vi "SERIAL_Close.vi"(11 "navX DevRef":T1={"SerialPortRef"={"DevStatus"={"status"=FALSE, "code"=0, "source"=""}, "Serial Port Name"=""}, "Board Information"={"WhoAmI (50 | 0x32)"=0, "Board Revision"=0, "Firmware Major Version"=0, "Firmware Minor Version"=0}, "Status"={"Update Rate Hz"=0, "Accelerometer Full-Scale Range"=0, "Gyro Full-Scale Range"=0, "NAVX_OP_STATUS"=0, "NAVX_CAL_STATUS"=0, "NAVX_SELFTEST_STATUS"=0, "NAVX_SENSOR_STATUS"={"MOVING"=FALSE, "YAW_STABLE"=FALSE, "MAG_DISTURBANCE"=FALSE, "ALTITUDE_VALID"=FALSE, "SEALEVEL_PRESS_SET"=FALSE, "FUSED_HEADING_VALID"=FALSE}}, "Offsets"={"Yaw"=0.0, "Quat W"=0.0, "Quat X"=0.0, "Quat Y"=0.0, "Quat Z"=0.0}, "Update Rate (4Hz-60Hz)"=50, "Nav6Mode (YPR)"=enum."YPR", "refnum name"="", "error"={"status"=FALSE, "code"=0, "source"=""}, "Loop VI Refnum"=refnum} {"Status"."NAVX_OP_STATUS" items=["INITIALIZING", "SELFTEST_IN_PROGRESS", "ERROR", "IMU_AUTOCAL_IN_PROGRESS", "NORMAL"]; "Status"."NAVX_CAL_STATUS" items=["IMU_CAL_STATE_MASK"=3, "IMU_CAL_INPROGRESS"=0, "IMU_CAL_ACCUMULATE"=1, "IMU_CAL_COMPLETE"=2, "MAG_CAL_COMPLETE"=4, "BARO_CAL_COMPLETE"=8]}) -> (0 "error out":errorcluster)   [LabVIEW 2014, in "navX-MXP IMU.lvlib"]
uses:
  navX-MXP IMU.lvlib
  Internal/navX Serial DevRef.ctl
  <vilib>/Rock Robotics/WPI/SerialPort/WPI_SerialPortRef.ctl
  COMMON/TypeDefs/Data TypeDefs/navX Board Information.ctl
  COMMON/TypeDefs/Data TypeDefs/navX Status Data.ctl
  COMMON/TypeDefs/Value TypeDefs/navX NAVX_OP_STATUS.ctl
  COMMON/TypeDefs/Value TypeDefs/navX NAVX_CAL_STATUS.ctl
  COMMON/TypeDefs/Value TypeDefs/navX NAVX_SENSOR_STATUS.ctl
  TypeDefs/navX Serial Mode.ctl
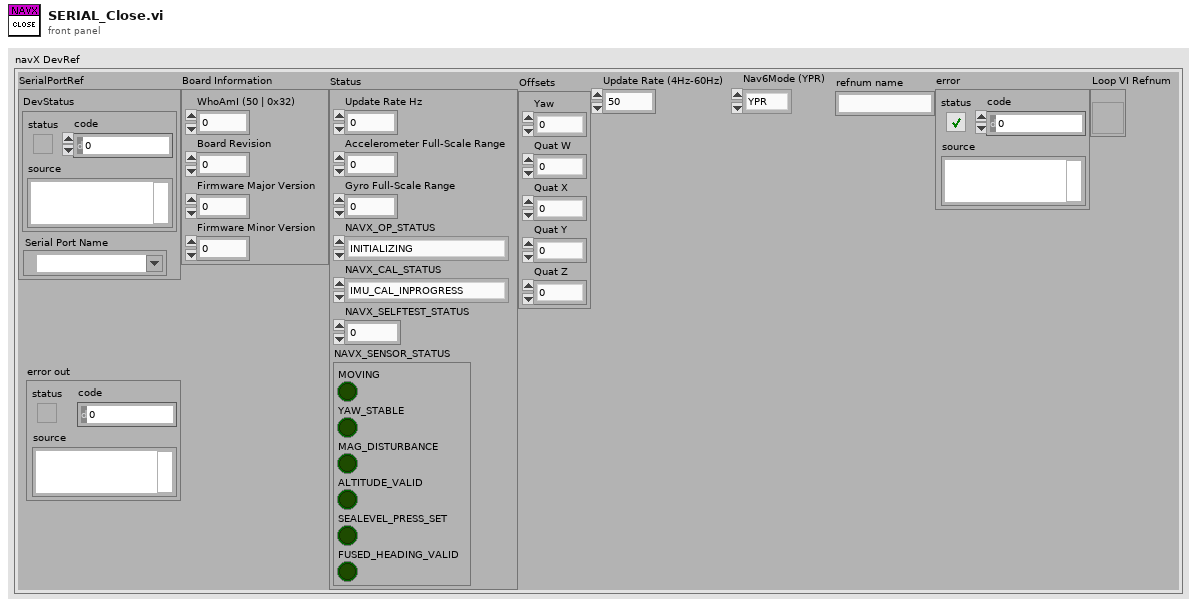
[diagram p1: front panel]
types:
  T1 = typedef "navX-MXP IMU.lvlib/navX Serial DevRef.ctl" = cluster{"SerialPortRef":T2, "Board Information":T3, "Status":T4, "Offsets":cluster{"Yaw":dbl, "Quat W":dbl, "Quat X":dbl, "Quat Y":dbl, "Quat Z":dbl}, "Update Rate (4Hz-60Hz)":u8, "Nav6Mode (YPR)":T8, "refnum name":string, "error":errorcluster, "Loop VI Refnum":refnum<vi>}
  T2 = typedef "WPI_SerialPortRef.ctl" = cluster{"DevStatus":errorcluster, "Serial Port Name":refnum<visa-resource-name>}
  T3 = typedef "navX-MXP IMU.lvlib/navX Board Information.ctl" = cluster{"WhoAmI (50 | 0x32)":u8, "Board Revision":u8, "Firmware Major Version":u8, "Firmware Minor Version":u8}
  T4 = typedef "navX-MXP IMU.lvlib/navX Status Data.ctl" = cluster{"Update Rate Hz":u8, "Accelerometer Full-Scale Range":u8, "Gyro Full-Scale Range":u16, "NAVX_OP_STATUS":T5, "NAVX_CAL_STATUS":T6, "NAVX_SELFTEST_STATUS":u8, "NAVX_SENSOR_STATUS":T7}
  T5 = typedef "navX-MXP IMU.lvlib/navX NAVX_OP_STATUS.ctl" = u8
  T6 = typedef "navX-MXP IMU.lvlib/navX NAVX_CAL_STATUS.ctl" = u8
  T7 = typedef "navX-MXP IMU.lvlib/navX NAVX_SENSOR_STATUS.ctl" = cluster{"MOVING":bool, "YAW_STABLE":bool, "MAG_DISTURBANCE":bool, "ALTITUDE_VALID":bool, "SEALEVEL_PRESS_SET":bool, "FUSED_HEADING_VALID":bool}
  T8 = typedef "navX-MXP IMU.lvlib/navX Serial Mode.ctl" = enum16{"YPR", "Gyro", "Quaternion"}
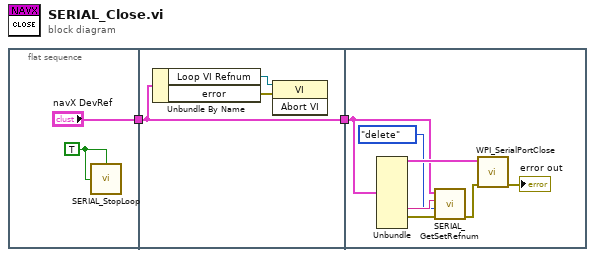
[diagram p0: block diagram]
diagram:
  n1 = flat-sequence {
    tunnel: ["navX DevRef"] -> w1
    tunnel: [w7] -> w2
    tunnel: w1 -> [w7]
    tunnel: w2 -> [w8]
    frame #0 {
      w4 = TRUE ("Stop?")
      n2 = call "SERIAL_StopLoop.vi"("Stop?"=w4, "Update?"=w4) -> ()  [unwired: 1 out]
    }
    frame #1 {
      n3 = Unbundle By Name(w7) -> ("Loop VI Refnum"=w6:refnum<vi>, "error"=w5:errorcluster)
      n4 = invoke class="VI" method="Abort VI"(reference=w6, error in=w5) -> ()  [unwired: 1 in, 3 out]
    }
    frame #2 {
      n5 = Unbundle(w8) -> ("SerialPortRef"=w14:T2, "refnum name"=w12:string, "error"=w10:errorcluster)  [unwired: 6 out]
      n6 = call "SERIAL_GetSetRefnum.vi"("error in (no error)"=w10, "menu"=enum16{"set", "get", "delete"}."delete", "refnum name"=w12, "navX DevRef"=w8) -> ("error out"=w9:errorcluster)  [unwired: 6 in, 1 out]
      n7 = call <vilib>:"WPI_SerialPortClose.vi"("error in (no error)"=w9, "SerialPortRef"=w14) -> ("error out"=→"error out":errorcluster)  [unwired: 9 in]
    }
  }
